vi "test2.vi"() -> ()   [LabVIEW 2018]
uses:
  <vilib>/imath/engines/lvmath/Plug In/_Char/NIMS_CH_character datatype.ctl
  <vilib>/imath/engines/lvmath2/RunTimeEngine/Managers/WorkSpace/UID Generator.vi
  <vilib>/imath/engines/lvmath/Plug In/_Char/NIMS_CH_Character RV to String.vi
  <vilib>/imath/engines/lvmath2/RunTimeEngine/BuiltInFunctions/random/NIMS_random.vi
  <vilib>/imathl/engines/lvmath/Functions/Error Handling/Create Error.vi
  <vilib>/imath/engines/lvmath2/RunTimeEngine/BuiltInFunctions/fir_win/NIMS_fir_win(I32,V,Str,V,Str).vi
  <vilib>/imath/engines/lvmath2/RunTimeEngine/ErrorHandling/NIMS_Create Error From Enums.vi
  <vilib>/imath/engines/lvmath2/RunTimeEngine/BuiltInFunctions/conv/NIMS_conv(M,M).vi
  <instcachedir>/0/NIMS_conv(M,M)_D972F9B3CDFC4C878A09791DEDB45279.lvgen/NIMS_conv(M,M)_D972F9B3CDFC4C878A09791DEDB45279_001.vi
  <vilib>/imath/engines/lvmath2/RunTimeEngine/ErrorHandling/NIMS_Error From Error Code.vi
  <vilib>/imath/engines/lvmath2/RunTimeSupport/NIMS_Get Any Vector_w Error - Matrix.vi
  <instcachedir>/0/NIMS_Get Any Vector_w Error - Matrix_1B26302039EC43C7B9FA287B1E12D88C.lvgen/NIMS_Get Any Vector_w Error - Matrix_1B26302039EC43C7B9FA287B1E12D88C_001.vi
  <vilib>/imath/engines/lvmath2/RunTimeEngine/BuiltInFunctions/psd_periodogram/NIMS_psd_periodogram().vi
  <instcachedir>/0/NIMS_psd_periodogram()_02030E41DB254B5B8F4838052F408B46.lvgen/NIMS_psd_periodogram()_02030E41DB254B5B8F4838052F408B46_000.vi
  <vilib>/imath/engines/lvmath2/RunTimeEngine/RunTimeType/NIMS_RunTimeType_From StrictType (excl LVString).vi
  <instcachedir>/0/NIMS_RunTimeType_From StrictType (excl LVString)_E7E34A65C99947108168652BAD14964D.lvgen/NIMS_RunTimeType_From StrictType (excl LVString)_E7E34A65C99947108168652BAD14964D_000.vi
  <vilib>/imath/engines/lvmath2/RunTimeEngine/LocalVariableDefStatement/MC_LocalVariableDefStatement_Display.vi
  <vilib>/imath/engines/lvmath2/RunTimeEngine/BuiltInFunctions/crosscorr/NIMS_crosscorr(GM,Str).vi
  <instcachedir>/0/NIMS_crosscorr(GM,Str)_B40E69E1A515490ABE9B33FB59F56A52.lvgen/NIMS_crosscorr(GM,Str)_B40E69E1A515490ABE9B33FB59F56A52_000.vi
  <vilib>/imath/engines/lvmath2/RunTimeEngine/BuiltInFunctions/hilbert/NIMS_hilbert(RM, I32).vi
  <vilib>/imath/engines/lvmath2/RunTimeEngine/BuiltInFunctions/imag/NIMS_imag(Complex).vi
  <instcachedir>/0/NIMS_imag(Complex)_3180D40D00C843A49C2B33397F857BF3.lvgen/NIMS_imag(Complex)_3180D40D00C843A49C2B33397F857BF3_001.vi
  <vilib>/imath/engines/lvmath2/RunTimeEngine/BuiltInFunctions/size/NIMS_[I32,I32]=size(GM).vi
  <instcachedir>/0/NIMS_[I32,I32]=size(GM)_B0A6EC1255BB4C8AB801FE6F734128D9.lvgen/NIMS_[I32,I32]=size(GM)_B0A6EC1255BB4C8AB801FE6F734128D9_000.vi
  <vilib>/imath/engines/lvmath2/RunTimeEngine/RangeToken/NIMS_Range.vi
  <instcachedir>/0/NIMS_Range_846134F467D14A349F7C6CCEF459CDB2.lvgen/NIMS_Range_846134F467D14A349F7C6CCEF459CDB2_000.vi
  <vilib>/imath/engines/lvmath2/RunTimeEngine/ArithmeticOperatorToken/NIMS_ArithmeticOperator_times.vi
  <instcachedir>/0/NIMS_ArithmeticOperator_times_D7E4A7A4AD2C4409A0CE309D2741A5B4.lvgen/NIMS_ArithmeticOperator_times_D7E4A7A4AD2C4409A0CE309D2741A5B4_007.vi
  <vilib>/imath/engines/lvmath2/RunTimeEngine/ArithmeticOperatorToken/NIMS_ArithmeticOperator_plus.vi
  <instcachedir>/0/NIMS_ArithmeticOperator_plus_DE670E32103C4C10ADF2A97367172B30.lvgen/NIMS_ArithmeticOperator_plus_DE670E32103C4C10ADF2A97367172B30_003.vi
  <vilib>/imath/engines/lvmath2/RunTimeEngine/ArithmeticOperatorToken/NIMS_ArithmeticOperator_minus.vi
  <instcachedir>/0/NIMS_ArithmeticOperator_minus_C4D0373119CC411691B2E50DF2E09F22.lvgen/NIMS_ArithmeticOperator_minus_C4D0373119CC411691B2E50DF2E09F22_002.vi
  <vilib>/imath/engines/lvmath2/RunTimeEngine/BuiltInFunctions/fft/NIMS_fft(GM).vi
  <instcachedir>/0/NIMS_fft(GM)_4D6538E03936427980510B9710B4978C.lvgen/NIMS_fft(GM)_4D6538E03936427980510B9710B4978C_000.vi
  <vilib>/imath/engines/lvmath2/RunTimeEngine/BuiltInFunctions/abs/NIMS_abs(signed).vi
  <instcachedir>/0/NIMS_abs(signed)_C4FCB8E6058B49B797C7C8D53CA5F6EC.lvgen/NIMS_abs(signed)_C4FCB8E6058B49B797C7C8D53CA5F6EC_003.vi
  <vilib>/imath/engines/lvmath2/RunTimeEngine/BuiltInFunctions/eps/NIMS_eps.vi
  <vilib>/imath/engines/lvmath2/RunTimeSupport/NIMS_Error if Not Equal.vi
  <instcachedir>/0/NIMS_Error if Not Equal_C77461FADD9B4AE6B0EA3ED6E3A6D94D.lvgen/NIMS_Error if Not Equal_C77461FADD9B4AE6B0EA3ED6E3A6D94D_001.vi
  <vilib>/imath/engines/lvmath2/RunTimeEngine/IndexRead/NIMS M(V).vi
  <instcachedir>/0/NIMS M(V)_948FAC22C1C943948B75DA6190348614.lvgen/NIMS M(V)_948FAC22C1C943948B75DA6190348614_005.vi
  <vilib>/imath/engines/lvmath2/RunTimeEngine/Managers/SymbolTable/Clear UID.vi
  <vilib>/imath/engines/lvmath2/RunTimeEngine/NodeEndStatement/NIMS_NodeEndStatement_Output.vi
  <instcachedir>/0/NIMS_NodeEndStatement_Output_53EC0D466D134D7ABD903AC30B43404B.lvgen/NIMS_NodeEndStatement_Output_53EC0D466D134D7ABD903AC30B43404B_003.vi
  <instcachedir>/0/NIMS_NodeEndStatement_Output_53EC0D466D134D7ABD903AC30B43404B.lvgen/NIMS_NodeEndStatement_Output_53EC0D466D134D7ABD903AC30B43404B_005.vi
  <instcachedir>/0/NIMS_NodeEndStatement_Output_53EC0D466D134D7ABD903AC30B43404B.lvgen/NIMS_NodeEndStatement_Output_53EC0D466D134D7ABD903AC30B43404B_002.vi
  <vilib>/imath/engines/lvmath2/RunTimeEngine/ErrorHandling/NIMS_Finalize Error.vi
  <vilib>/imath/engines/lvmath2/RunTimeEngine/Managers/SymbolTable/NIMS_WorkSpace.lvlib
panel:
  out "低频过程As(t)样本的功率谱密度":cluster{"Y":dbl[], "Y":dbl[]}[](graph)
  out "低频过程Ac(t)样本的功率谱密度":cluster{"Y":dbl[], "Y":dbl[]}[](graph)
  out "低频过程As(t)样本的自相关函数":dbl[][](graph)
  out "窄带随机信号样本的功率谱密度":cluster{"Y":dbl[], "Y":dbl[]}[](graph)
  out "低频过程Ac(t)样本的自相关函数":dbl[][](graph)
  out "窄带随机信号样本的自相关函数":dbl[][](graph)
  out "As(t)时域波形":dbl[][](graph)
  out "Ac(t)时域波形":dbl[][](graph)
  out "窄带信号自相关函数":cluster{"Y":dbl[], "Y":dbl[]}[](graph)
  out "?":dbl[](graph)
  out "时域波形":dbl[][](graph)
  in  "M":dbl=200.0
  in  "fs":dbl=22000.0
  in  "deltf":dbl=500.0
  in  "f0":dbl=10000.0
  in  "N":dbl=10000.0
  # "窄带信号功率谱密度"
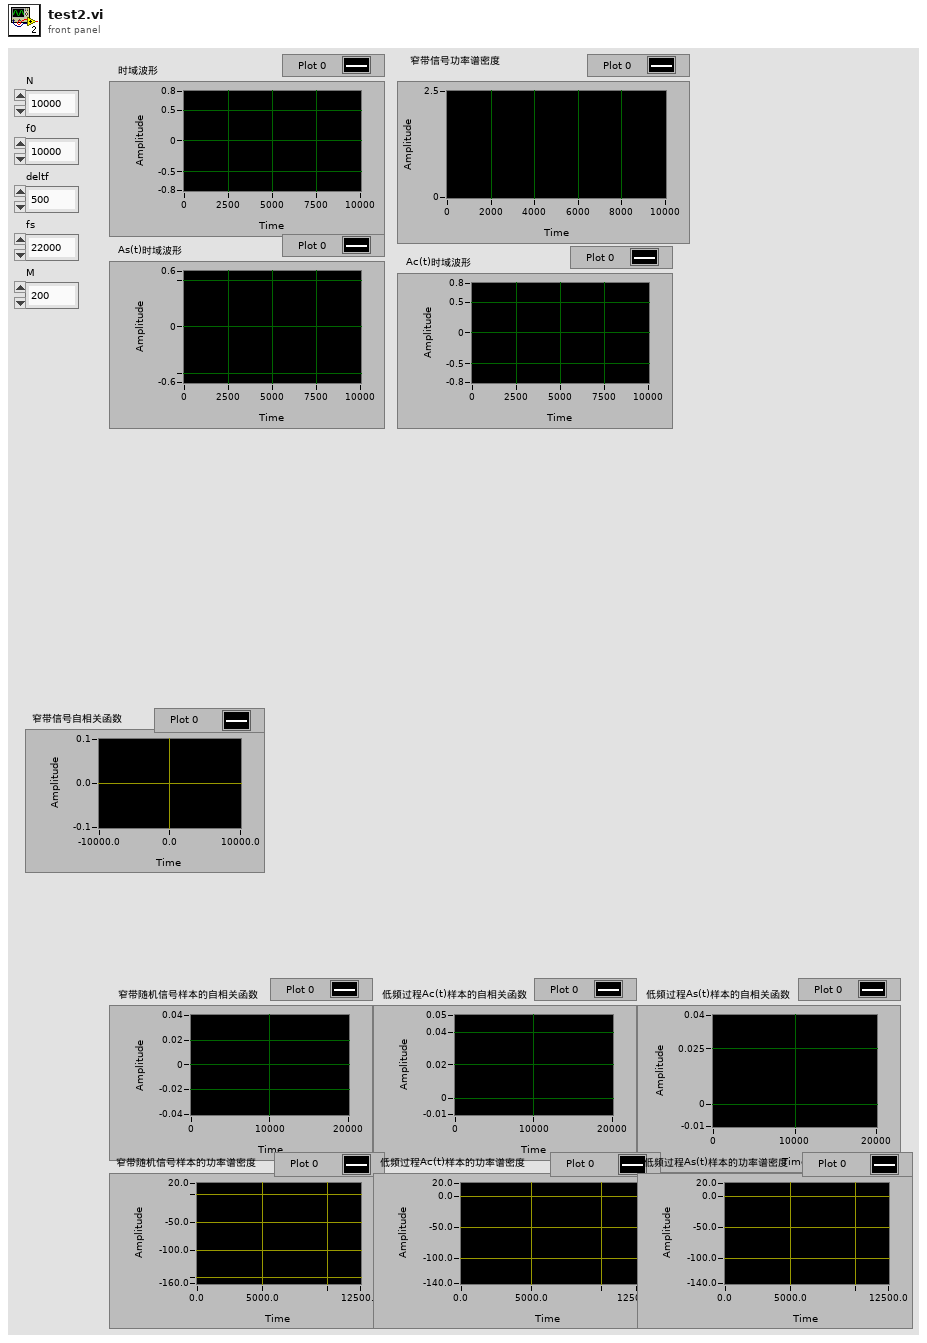
[diagram p1: front panel]
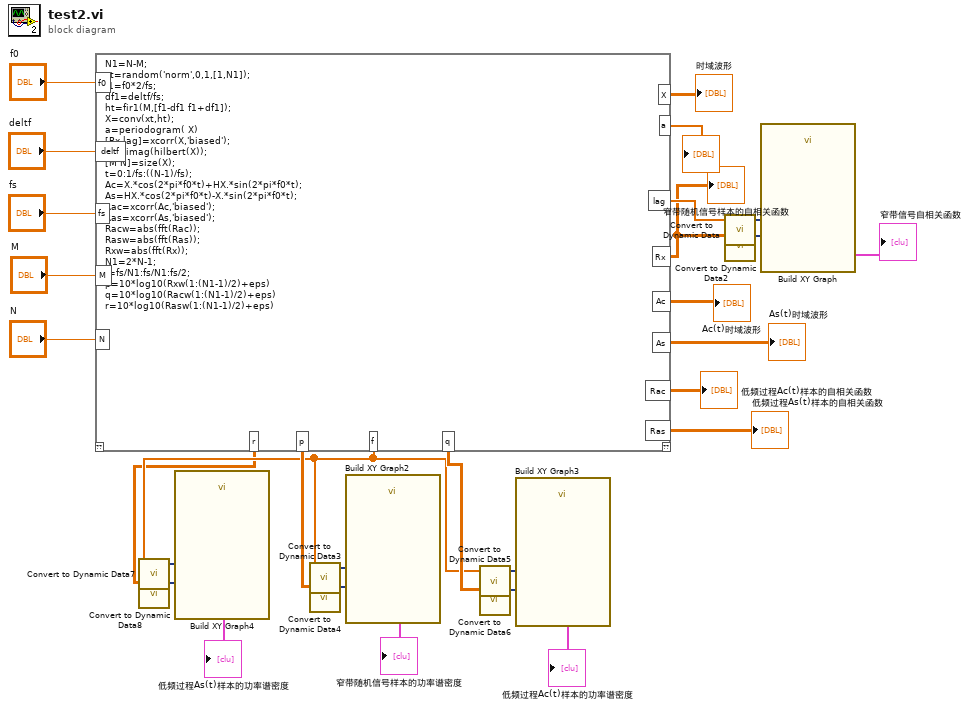
[diagram p0: block diagram]
diagram:
  n1 = mathscript code="N1=N-M;\nxt=random('norm',0,1,[1,N1]);\nf1=f0*2/fs;\ndf1=deltf/fs;\nht=fir1(M,[f1-df1 f1+df1]);\nX=conv(xt,ht);\na=periodogram( X)\n[Rx,lag]=xcorr(X,'biased');\nHX=imag(hilbert(X));\n[M N]=size(X);\nt=0:1/fs:((N-1)/fs);\nAc=X.*cos(2*pi*f0*t)+HX.*sin(2*pi*f0*t);\nAs=HX.*cos(2*pi*f0*t)-X.*sin(2*pi*f0*t);\nRac=xcorr(Ac,'biased');\nRas=xcorr(As,'biased'); \nRacw=abs(fft(Rac));\nRasw=abs(fft(Ras)); \nRxw=abs(fft(Rx));   \nN1=2*N-1;\nf=fs/N1:fs/N1:fs/2;  \np=10*log10(Rxw(1:(N1-1)/2)+eps)\nq=10*log10(Racw(1:(N1-1)/2)+eps)\nr=10*log10(Rasw(1:(N1-1)/2)+eps)"("f0"="f0", "deltf"="deltf", "fs"="fs", "M"="M", "N"="N") -> ("X"=→"时域波形":dbl[][], "a"=→"?":dbl[], "lag"=w21:dbl[], "Rx"=w13:dbl[][], "Ac"=→"Ac(t)时域波形":dbl[][], "As"=→"As(t)时域波形":dbl[][], "Rac"=→"低频过程Ac(t)样本的自相关函数":dbl[][], "Ras"=→"低频过程As(t)样本的自相关函数":dbl[][], "f"=w3:dbl[], "p"=w8:cdb[][], "q"=w5:cdb[][], "r"=w1:cdb[][])  [unwired: 1 in, 1 out]
  "窄带随机信号样本的自相关函数" <- w13
  n2 = call "Convert to Dynamic Data7"("Array"=w3) -> ("Dynamic Data Type"=w4:dynamicdata)  [unwired: 3 in]
  n3 = call "Convert to Dynamic Data8"("2D Array"=w1) -> ("Dynamic Data Type"=w2:dynamicdata)  [unwired: 3 in]
  n4 = call "Build XY Graph4"("Y Input"=w2, "X Input"=w4) -> ("XY Graph"=→"低频过程As(t)样本的功率谱密度":cluster{"X":dbl[], "Y":dbl[]}[])  [unwired: 8 in, 1 out]
  n5 = call "Convert to Dynamic Data3"("Array"=w3) -> ("Dynamic Data Type"=w10:dynamicdata)  [unwired: 3 in]
  n6 = call "Convert to Dynamic Data4"("2D Array"=w8) -> ("Dynamic Data Type"=w9:dynamicdata)  [unwired: 3 in]
  n7 = call "Build XY Graph2"("Y Input"=w9, "X Input"=w10) -> ("XY Graph"=→"窄带随机信号样本的功率谱密度":cluster{"X":dbl[], "Y":dbl[]}[])  [unwired: 8 in, 1 out]
  n8 = call "Convert to Dynamic Data5"("Array"=w3) -> ("Dynamic Data Type"=w7:dynamicdata)  [unwired: 3 in]
  n9 = call "Convert to Dynamic Data6"("2D Array"=w5) -> ("Dynamic Data Type"=w6:dynamicdata)  [unwired: 3 in]
  n10 = call "Build XY Graph3"("Y Input"=w6, "X Input"=w7) -> ("XY Graph"=→"低频过程Ac(t)样本的功率谱密度":cluster{"X":dbl[], "Y":dbl[]}[])  [unwired: 8 in, 1 out]
  n11 = call "Convert to Dynamic Data"("Array"=w21) -> ("Dynamic Data Type"=w20:dynamicdata)  [unwired: 3 in]
  n12 = call "Convert to Dynamic Data2"("2D Array"=w13) -> ("Dynamic Data Type"=w19:dynamicdata)  [unwired: 3 in]
  n13 = call "Build XY Graph"("Y Input"=w19, "X Input"=w20) -> ("XY Graph"=→"窄带信号自相关函数":cluster{"X":dbl[], "Y":dbl[]}[])  [unwired: 8 in, 1 out]
